vi "HexCenterFinder4Sides.vi"() -> ()   [LabVIEW 2019]
panel:
  in  "SiOnBP?":bool
  out "zAvg":dbl
  out "Output XYZU":string
  out "x":dbl
  out "y":dbl
  out "Orinetation":dbl
  out "Intercepts":dbl[][](array[numeric])
  out "Angles":dbl[][](array[numeric])
  out "Slopes":dbl[][](array[numeric])
  out "S1":T1(plugin-control)
  in  "PCBEdges":path=path "C:/Users/TTUHEP/Documents/LabVIEW/Data/AssemblyIO_logs/PCBDefaultEdges.txt"
  in  "SiEdges":path=path "C:/Users/TTUHEP/Documents/LabVIEW/Data/AssemblyIO_logs/SiDefaultEdges.txt"
  in  "Component":enum16{"Baseplate", "Si", "PCB"}(ring)
  in  "BasePlateEdges":path=path "C:/Users/TTUHEP/Documents/LabVIEW/Data/AssemblyIO_logs/BasePlateDefaultEdges.txt"
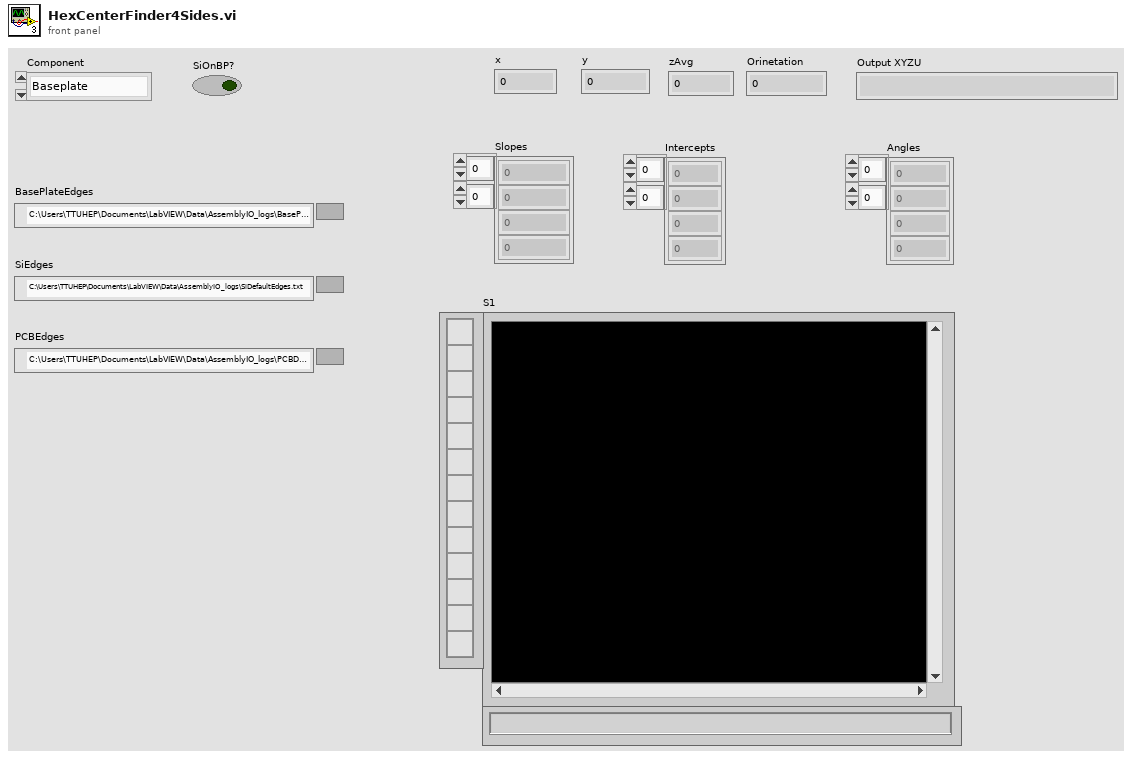
[diagram p1: front panel]
types:
  T1 = typedef "IMAQ Image.ctl" = refnum<image>
  T2 = typedef "IMAQ Line" = cluster{"Start X":i32, "Start Y":i32, "End X":i32, "End Y":i32}
  T3 = enum16{"Left Button", "Center Button", "Right Button", "Window Close"}
  T4 = enum16{"open", "replace", "create", "open or create", "replace or create", "replace or create with confirmation"}
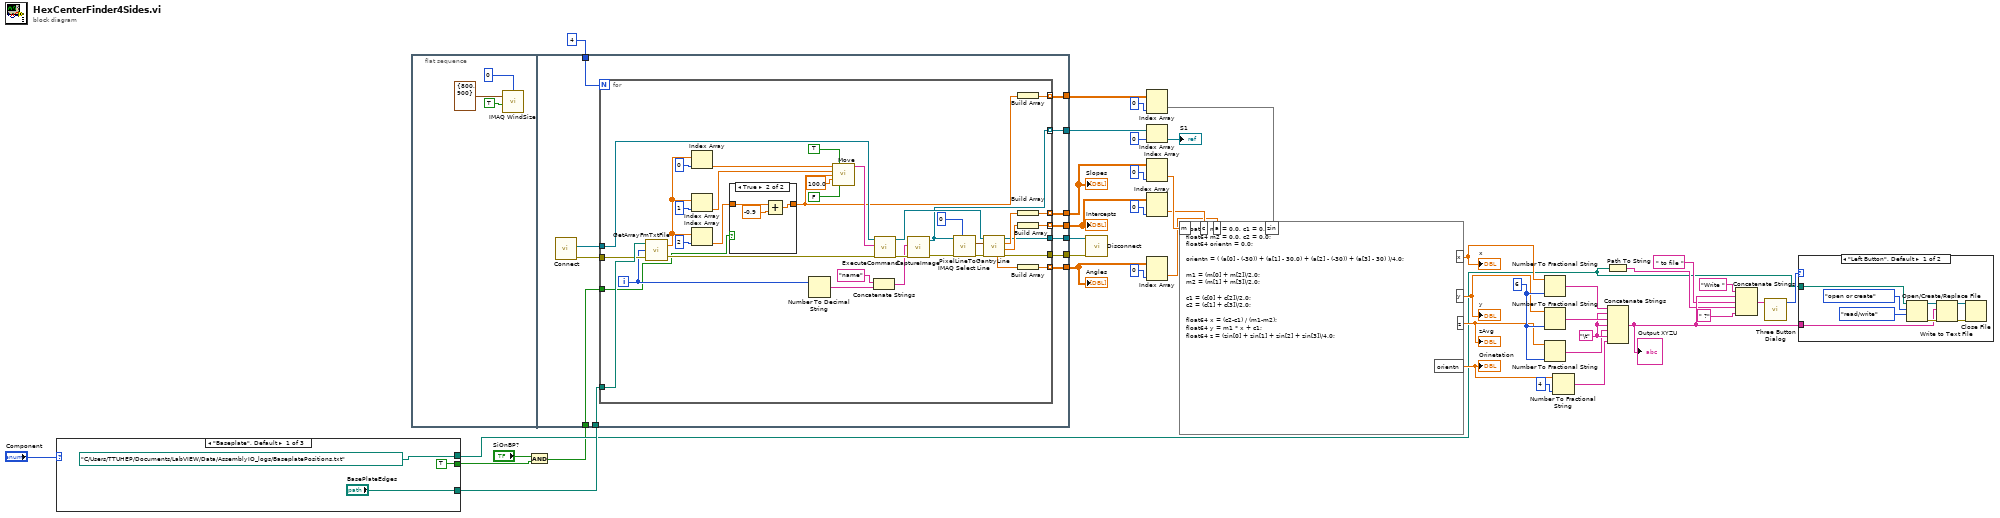
[diagram p0: block diagram]
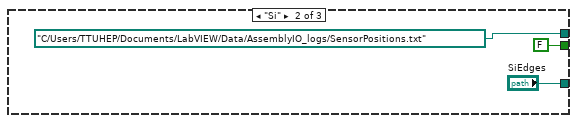
[diagram p4: hidden frame]
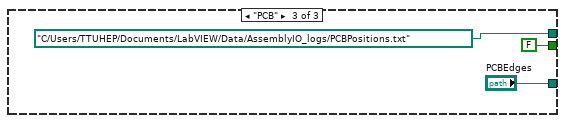
[diagram p5: hidden frame]
diagram:
  w23 = "\t"
  w16 = i16 6 ("width (-)")
  n1 = case shown="\"Baseplate\", Default" "Component" {
    tunnel: ["BasePlateEdges" "SiEdges" "PCBEdges"] -> w26
    tunnel: [path "C:/Users/TTUHEP/Documents/LabVIEW/Data/AssemblyIO_logs/BaseplatePositions.txt" ("OutFile") path "C:/Users/TTUHEP/Documents/LabVIEW/Data/AssemblyIO_logs/SensorPositions.txt" ("OutFile") path "C:/Users/TTUHEP/Documents/LabVIEW/Data/AssemblyIO_logs/PCBPositions.txt" ("OutFile")] -> w4
    tunnel: [TRUE ("y") FALSE ("y") FALSE ("y")] -> w3
    frame "Baseplate", Default {
    }
    frame "Si" {
    }
    frame "PCB" {
    }
  }
  n2 = flat-sequence {
    tunnel: 4 -> [w66]
    tunnel: w26 -> [w65]
    tunnel: [w64] -> w41
    tunnel: [w63] -> w40
    tunnel: [w62] -> w34
    tunnel: [w61] -> w31
    tunnel: [w60] -> w28
    tunnel: [w57] -> w39
    tunnel: [w56] -> w18
    tunnel: w1 -> [w55]
    frame #0 {
      n3 = call "IMAQ WindSize"("Scrollbars? (N)"=TRUE, "Width & Height"=cluster{"Width":i32, "Height":i32} {"Width"=800, "Height"=900}, "Window Number"=0) -> ()  [unwired: 3 in, 3 out]
    }
    frame #1 {
      n4 = call "Connect.vi"() -> ("error out"=w59:errorcluster, "controller"=w58:refnum<k24>)  [unwired: 10 in]
      n5 = for {
        N: w66 -> [_]
        tunnel: w65 -> [w99]
        tunnel: w58 -> [w83]
        tunnel: w59 -> [w82]
        tunnel: [w76] -> w64
        tunnel: [w75] -> w63
        tunnel: [w74] -> w62 mode=indexing
        tunnel: [w73] -> w61 mode=indexing
        tunnel: [w72] -> w60 mode=indexing
        tunnel: [w71] -> w57 mode=indexing
        tunnel: [w70] -> w56 mode=indexing
        tunnel: w55 -> [w69]
        i -> [w80]
        n6 = call "GetArrayFmTxtFile.vi"("error in"=w82, "LineNo."=w80, "TextFile"=w99) -> ("error out"=w81:errorcluster, "Array"=w100:dbl[])
        n7 = Index Array(array=w100, index=0) -> (element=w95:dbl)
        n8 = Index Array(array=w100, index=1) -> (element=w94:dbl)
        n9 = Index Array(array=w100, index=2) -> (element=w68:dbl)
        n10 = case shown="True" w69 {
          tunnel: w68 -> [w104 w107]
          tunnel: [w104 w105] -> w67
          frame False {
          }
          frame True {
            n11 = Add(x=w107, y=-0.9) -> (x+y=w105:dbl)
          }
        }
        n12 = Number To Decimal String(number=w80) -> (decimal integer string=w79:string)  [unwired: 1 in]
        n13 = call "Move.vi"("X"=w95, "Absolute"=TRUE, "Y"=w94, "Z"=w67, "SpeedXY (mm/s)"=100.0, "Move Z first"=FALSE) -> ("Position Gcode"=w84:string)  [unwired: 9 in]
        n14 = Concatenate Strings("name" ("string"), w79) -> (w77:string)
        n15 = call "ExecuteCommand.vi"("error in (no error)"=w81, "Command Code"=w84, "controller in"=w83) -> ("error out"=w93:errorcluster, "controller out"=w90:refnum<k24>)  [unwired: 6 in, 1 out]
        n16 = call "CaptureImage.vi"("ImageName"=w77, "error in (no error)"=w93) -> ("Image"=w71:T1, "error out"=w91:errorcluster)  [unwired: 5 in]
        n17 = call "IMAQ Select Line"("Window Number (0...15)"=0, "error in (no error)"=w91, "Image In"=w71) -> ("error out"=w88:errorcluster, "Line"=w89:T2)  [unwired: 5 in, 2 out]
        n18 = call "PixelLineToGantryLine.vi"("error in"=w88, "cluster"=w89, "Controller In"=w90) -> ("error out"=w76:errorcluster, "intercept"=w86:dbl, "slope"=w87:dbl, "controller out"=w75:refnum<k24>, "Angle(degree)"=w85:dbl)  [unwired: 4 in]
        n19 = Build Array(w67) -> (w70:dbl[])
        n20 = Build Array(w87) -> (w74:dbl[])
        n21 = Build Array(w86) -> (w73:dbl[])
        n22 = Build Array(w85) -> (w72:dbl[])
      }
    }
  }
  n23 = And(x="SiOnBP?", y=w3) -> (x .and. y?=w1:bool)
  n24 = call "Disconnect.vi"("error in (no error)"=w41, "controller"=w40) -> ()  [unwired: 9 in, 1 out]
  n25 = Index Array(array=w18, index (col)=0 ("disabled index (col)")) -> (element=w17:dbl[])  [unwired: 1 in]
  n26 = Index Array(array=w39, index=0) -> (element=→"S1":T1)
  n27 = Index Array(array=w34, index (col)=0 ("disabled index (col)")) -> (element=w35:dbl[])  [unwired: 1 in]
  n28 = Index Array(array=w31, index (col)=0 ("disabled index (col)")) -> (element=w30:dbl[])  [unwired: 1 in]
  n29 = Index Array(array=w28, index (col)=0 ("disabled index (col)")) -> (element=w27:dbl[])  [unwired: 1 in]
  n30 = formula code="float64 m1 = 0.0, c1 = 0.0;\nfloat64 m2 = 0.0, c2 = 0.0;\nfloat64 orientn = 0.0;\n\norientn = ( (a[0] - (-30)) + (a[1] - 30.0) + (a[2] - (-30)) + (a[3] - 30) )/4.0;\n\nm1 = (m[0] + m[2])/2.0;\nm2 = (m[1] + m[3])/2.0;\n\nc1 = (c[0] + c[2])/2.0;\nc2 = (c[1] + c[3])/2.0;\n\nfloat64 x = (c2-c1) / (m1-m2);\nfloat64 y = m1 * x + c1;\nfloat64 z = (zin[0] + zin[1] + zin[2] + zin[3])/4.0;"("m"=w35, "c"=w30, "a"=w27, "zin"=w17) -> ("orientn"=w20:dbl, "x"=w6:dbl, "y"=w5:dbl, "z"=w15:dbl)
  "Orinetation" <- w20
  "y" <- w5
  "x" <- w6
  "zAvg" <- w15
  n31 = Number To Fractional String(number=w6, precision (6)=w16) -> (F-format string=w25:string)  [unwired: 2 in]
  n32 = Number To Fractional String(number=w5, precision (6)=w16) -> (F-format string=w24:string)  [unwired: 2 in]
  n33 = Number To Fractional String(number=w15, precision (6)=w16) -> (F-format string=w14:string)  [unwired: 2 in]
  n34 = Number To Fractional String(number=w20, precision (6)=i16 4 ("width (-)")) -> (F-format string=w21:string)  [unwired: 2 in]
  n35 = Path To String(path=w4) -> (string=w10:string)
  n36 = Concatenate Strings(w25, w23, w24, w23, w14, w23, w21) -> (w12:string)
  "Output XYZU" <- w12
  n37 = Concatenate Strings("Write ", w12, " to file ", w10, " ?" ("string")) -> (w8:string)
  n38 = call <vilib>:"Three Button Dialog.vi"("message"=w8) -> ("Which Button?"=w7:T3)  [unwired: 10 in]
  n39 = case shown="\"Left Button\", Default" w7 {
    tunnel: w12 -> [w109 _]
    tunnel: w4 -> [w108 _]
    frame "Left Button", Default {
      n40 = Open/Create/Replace File(file path (use dialog)=w108, operation (0:open)=T4."open or create", access (0:read/write)=enum16{"read/write", "read-only", "write-only"}."read/write") -> (refnum out=w115:refnum<file>, error out=w112:errorcluster)  [unwired: 3 in, 1 out]
      n41 = Write to Text File(file (use dialog)=w115, text=w109, error in=w112) -> (refnum out=w110:refnum<file>, error out=w111:errorcluster)  [unwired: 1 in, 1 out]
      n42 = Close File(refnum=w110, error in=w111) -> ()  [unwired: 2 out]
    }
    frame "Center Button" {
    }
  }
  "Slopes" <- w34
  "Angles" <- w28
  "Intercepts" <- w31
